vi "pict.GenColours.greyscale.vi"() -> (1 "colours":u32[](array[numeric]) format="%06x")   [LabVIEW 2020]
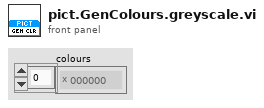
[diagram p1: front panel]
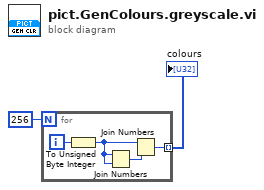
[diagram p0: block diagram]
diagram:
  n1 = for {
    N: 256 -> [_]
    tunnel: [w4] -> w2 mode=indexing
    i -> [w6]
    n2 = To Unsigned Byte Integer(number=w6) -> (unsigned 8bit integer=w3:u8)
    n3 = Join Numbers(hi=w3, lo=w3) -> ((hi.lo)=w5:u16)
    n4 = Join Numbers(hi=w3, lo=w5) -> ((hi.lo)=w4:u32)
  }
  "colours" <- w2
